vi "Configure File Extension.vi"(8 "Error In":errorcluster, 11 "File Extension":string="csv") -> (0 "Error Out":errorcluster)   [LabVIEW 2018, in "Toolkit.lvlib"]
doc: "Changes the default log file extension. The default is \"csv\"."
uses:
  Toolkit.lvlib
  Support/File/File Action.ctl
  Support/File/File.lvlib
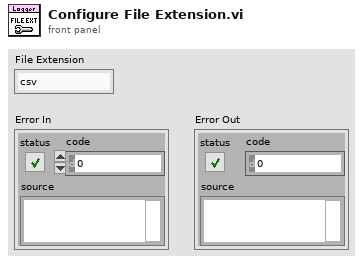
[diagram p1: front panel]
types:
  T1 = typedef "Toolkit.lvlib/File.lvlib/File Action.ctl" = enum16{"Initialize", "Set Maximum File Size", "Set Maximum File Count", "Set Root Folder", "Set Enable Calendar Folder Tree", "Set File Extension", "Start", "Write", "Stop", "Shutdown"}
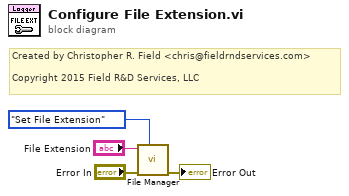
[diagram p0: block diagram]
diagram:
  # "Created by Christopher R. Field <chris@fieldrndservices.com>\n\nCopyright 2015 Field R&D Services, LLC"
  n1 = call "File Manager.vi"("Action"=File_Action."Set File Extension", "Error In"="Error In", "Set Value"="File Extension") -> ("Error Out"=→"Error Out":errorcluster)  [unwired: 8 in]
